vi "Array Functions Part 3.vi"() -> ()   [LabVIEW 2015]
panel:
  out "reversed array":string[](array[string])
  out "index of element - not found":i32
  out "sorted array":string[](array[string])
  out "index of element":i32
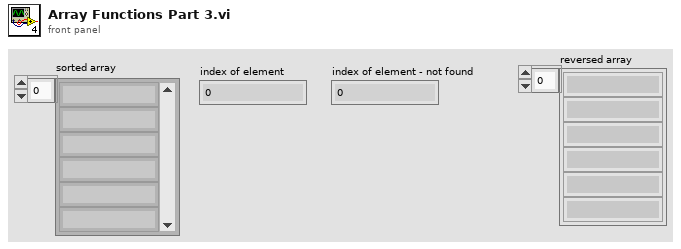
[diagram p1: front panel]
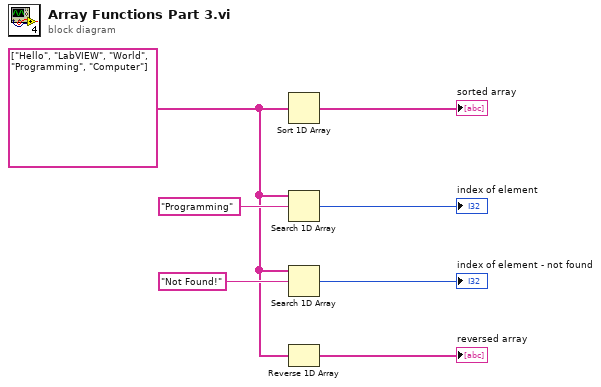
[diagram p0: block diagram]
diagram:
  w2 = string[] ["Hello", "LabVIEW", "World", "Programming", "Computer"]
  n1 = Sort 1D Array(array=w2) -> (sorted array=→"sorted array":string[])
  n2 = Search 1D Array(1D array=w2, element="Programming" ("String")) -> (index of element=→"index of element":i32)  [unwired: 1 in]
  n3 = Search 1D Array(1D array=w2, element="Not Found!" ("String")) -> (index of element=→"index of element - not found":i32)  [unwired: 1 in]
  n4 = Reverse 1D Array(array=w2) -> (reversed array=→"reversed array":string[])
